vi "StartAcquisition.vi"(8 "error in (no error)":errorcluster, 11 "reference in":refnum<class "Camera_IMAQdx.lvclass">) -> (0 "error out":errorcluster, 3 "reference out":refnum<class "Camera_IMAQdx.lvclass">)   [LabVIEW 2017, in "Camera_IMAQdx.lvclass"]
doc: "Starts IMAQdx Acquisition. Use this with Grab."
uses:
  Camera_IMAQdx.lvclass
  <vilib>/vision/driver/IMAQdx.llb/IMAQdx Acquisition Mode.ctl
  <vilib>/vision/driver/NI_Vision_Acquisition_Software.lvlib
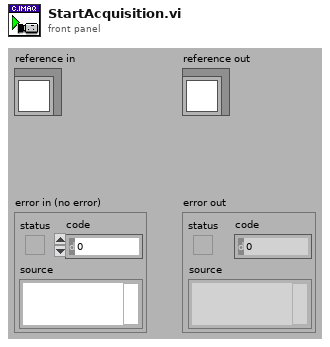
[diagram p1: front panel]
types:
  T1 = typedef "NI_Vision_Acquisition_Software.lvlib/IMAQdx Acquisition Mode.ctl" = enum32{"One Shot", "Continuous"}
  T2 = typedef "Camera_IMAQdx.lvclass/Configuration--Cluster.ctl" = cluster{"Camera Interface Name":string, "Number of Buffers":u32, "Image Name":string, "Image Type":T3}
  T3 = typedef "Image Type" = u32
  T4 = typedef "IMAQdx.ctl" = refnum<k21>
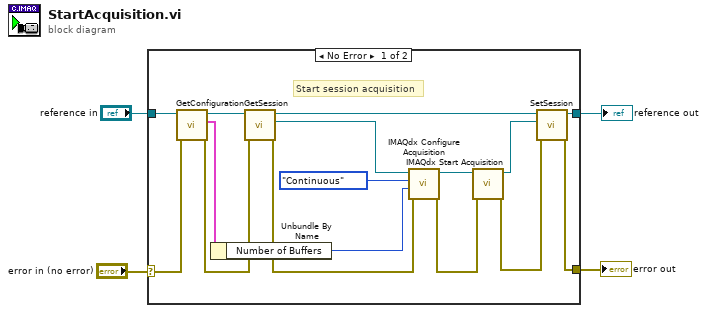
[diagram p0: block diagram]
diagram:
  n1 = case shown="No Error" "error in (no error)" {
    selector: "error in (no error)" -> [w14 w22]
    tunnel: [w5 w22] -> w3
    tunnel: [w8 w21] -> w1
    tunnel: "reference in" -> [w20 w21]
    frame No Error {
      # "Start session acquisition"
      n2 = call-dynamic "GetConfiguration.vi"("error in (no error)"=w14, "reference in"=w20) -> ("error out"=w13:errorcluster, "Configuration"=w12:T2, "reference out"=w15:refnum<class "Camera_IMAQdx.lvclass">)  [unwired: 7 in]
      n3 = Unbundle By Name(w12) -> ("Number of Buffers"=w11:u32)
      n4 = call "GetSession.vi"("error in (no error)"=w13, "reference in"=w15) -> ("error out"=w10:errorcluster, "Session"=w18:T4, "reference out"=w19:refnum<class "Camera_IMAQdx.lvclass">)  [unwired: 7 in]
      n5 = call <vilib>:"IMAQdx Configure Acquisition.vi"("error in"=w10, "Number of Buffers"=w11, "Continuous?"=IMAQdx_Acquisition_Mode."Continuous", "Session In"=w18) -> ("error out"=w9:errorcluster, "Session Out"=w17:T4)  [unwired: 6 in]
      n6 = call <vilib>:"IMAQdx Start Acquisition.vi"("error in"=w9, "Session In"=w17) -> ("error out"=w6:errorcluster, "Session Out"=w7:T4)  [unwired: 8 in]
      n7 = call "SetSession.vi"("error in (no error)"=w6, "Session"=w7, "reference in"=w19) -> ("error out"=w5:errorcluster, "reference out"=w8:refnum<class "Camera_IMAQdx.lvclass">)  [unwired: 7 in]
    }
    frame Error {
    }
  }
  "error out" <- w3
  "reference out" <- w1
